vi "PH_Stepmotor_BaseClass.PC Write PSDB.vi"(0 "i ref in":refnum<vi>, 5 "error IO":errorcluster) -> (14 "i ref out":refnum<vi>, 19 "error out":errorcluster)   [LabVIEW 2014, in "PH_Stepmotor_BaseClass.lvlib"]
doc: "This is the proc case which writes data to the PHELIX shot data base."
uses:
  PH_Stepmotor_BaseClass.lvlib
  PH_PSDBWriter/PH_PSDBWriter.lvlib
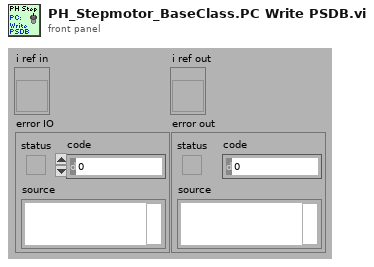
[diagram p1: front panel]
types:
  T1 = typedef "PH_PSDBWriter.lvlib/PH_PSDBWriter.Boolean dataset.ctl" = cluster{"name":string, "data":bool, "unit":string}
  T2 = typedef "PH_PSDBWriter.lvlib/PH_PSDBWriter.Numeric dataset.ctl" = cluster{"name":string, "data":dbl, "unit":string}
  T3 = typedef "PH_PSDBWriter.lvlib/PH_PSDBWriter.String dataset.ctl" = cluster{"name":string, "data":string, "unit":string}
  T4 = typedef "PH_PSDBWriter.lvlib/PH_PSDBWriter.PSDB Dataset.ctl" = cluster{"Version":i32, "2D data Input":T5[], "Boolean Input":T1[], "Image Input":T7[], "Numeric Input":T2[], "String Input":T3[]}
  T5 = typedef "PH_PSDBWriter.lvlib/PH_PSDBWriter.2D dataset.ctl" = cluster{"name":string, "data":dbl[][], "axis description":T6}
  T6 = typedef "PSDB.lvlib/PSDB_AxisDescription.ctl" = cluster{"x axis label":string, "y axis label":string, "x axis unit":string, "y axis unit":string}
  T7 = typedef "PH_PSDBWriter.lvlib/PH_PSDBWriter.Image dataset.ctl" = cluster{"name":string, "data":T8, "unit":string}
  T8 = typedef "IMAQ Image.ctl" = refnum<image>
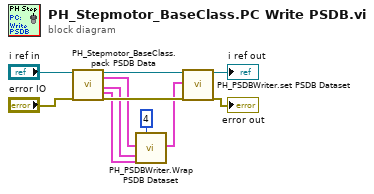
[diagram p0: block diagram]
diagram:
  n1 = call "PH_Stepmotor_BaseClass.pack PSDB Data.vi"("i ref in"="i ref in", "error in (no error)"="error IO") -> ("VI out"=w8:refnum<vi>, "PSDB Boolean Data Array"=w1:T1[], "PSDB Numeric Data Array"=w3:T2[], "PSDB String Data Array"=w4:T3[], "error out"=w10:errorcluster)  [unwired: 13 in]
  n2 = call "PH_PSDBWriter.Wrap PSDB Dataset.vi"("Version"=4, "Boolean Input"=w1, "Numeric Input"=w3, "String Input"=w4) -> ("PSDB Dataset"=w5:T4)  [unwired: 15 in]
  n3 = call "PH_PSDBWriter.set PSDB Dataset.vi"("VI in"=w8, "PSDB Dataset"=w5, "error in (no error)"=w10) -> ("VI out"=→"i ref out":refnum<vi>, "error out"=→"error out":errorcluster)  [unwired: 15 in]
